vi "OEE_SCREEN_1_recolor_init.vi"(7 "SCREEN_1_recolor_references":T1, 8 "error_in":errorcluster) -> (0 "error_out":errorcluster)   [LabVIEW 2019]
uses:
  typedef/SCREEN_1_recolor_references.ctl
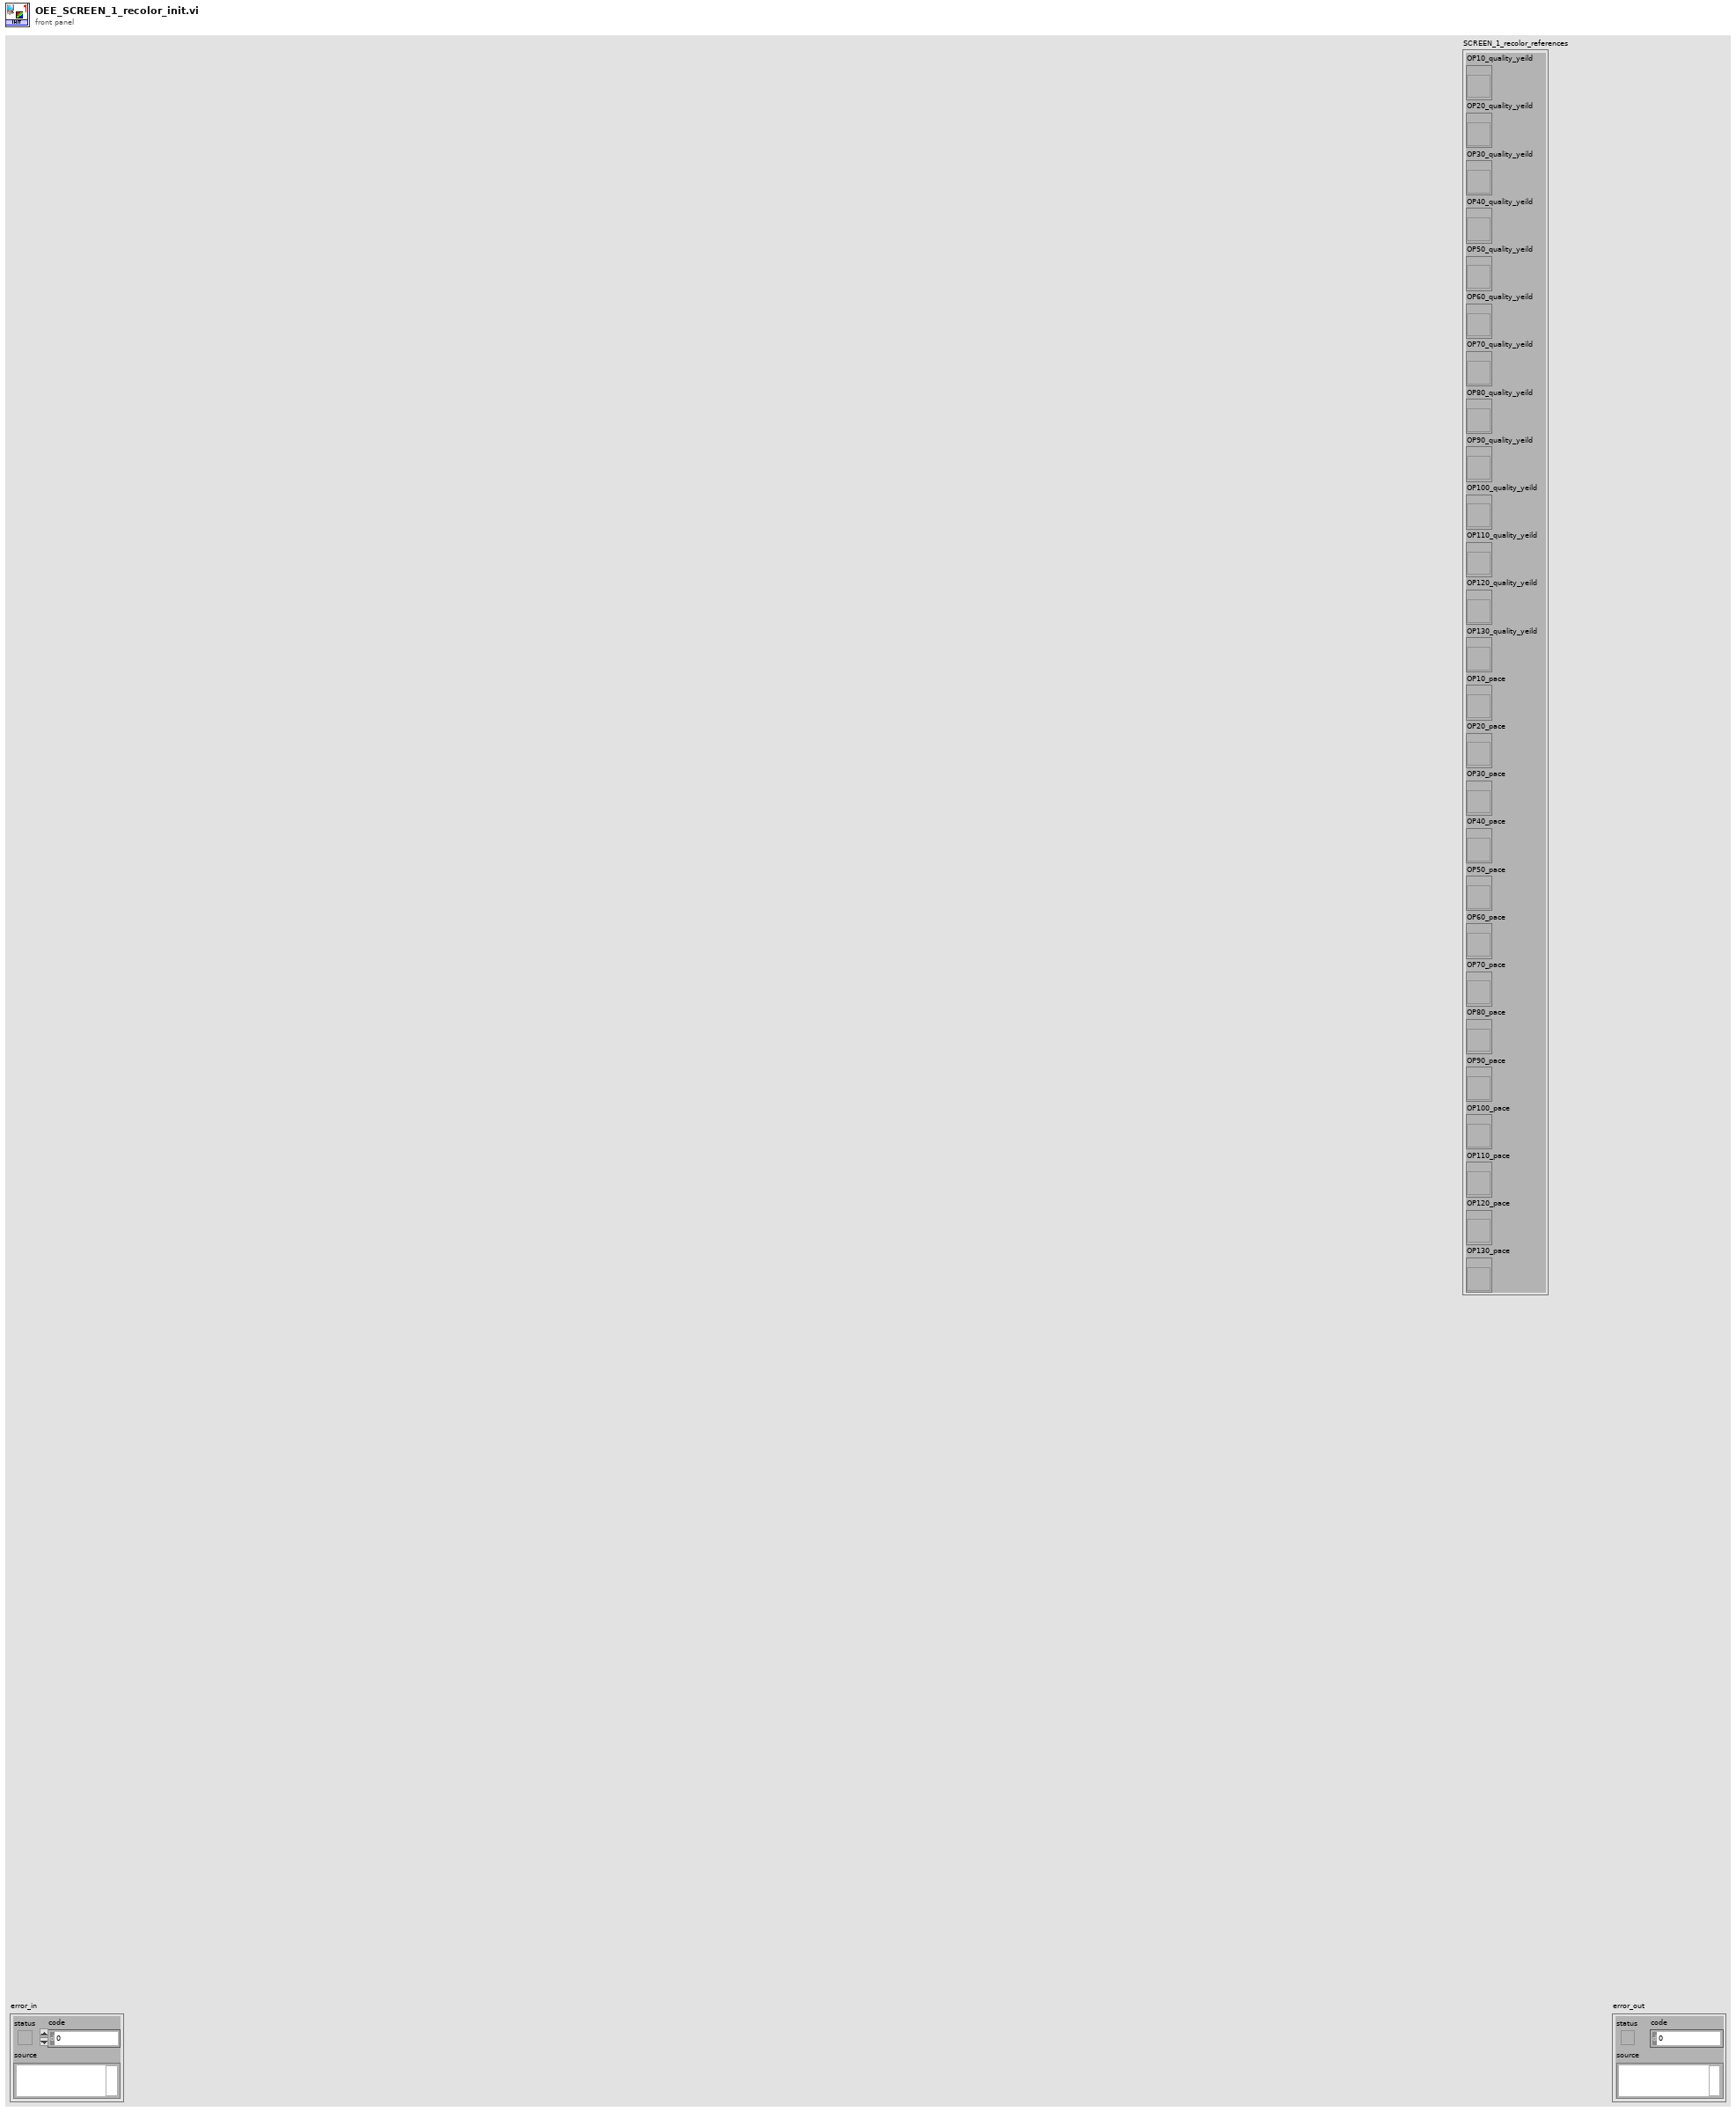
[diagram p1: front panel]
types:
  T1 = typedef "SCREEN_1_recolor_references.ctl" = cluster{"OP10_quality_yeild":refnum<vi>, "OP20_quality_yeild":refnum<vi>, "OP30_quality_yeild":refnum<vi>, "OP40_quality_yeild":refnum<vi>, "OP50_quality_yeild":refnum<vi>, "OP60_quality_yeild":refnum<vi>, "OP70_quality_yeild":refnum<vi>, "OP80_quality_yeild":refnum<vi>, "OP90_quality_yeild":refnum<vi>, "OP100_quality_yeild":refnum<vi>, "OP110_quality_yeild":refnum<vi>, "OP120_quality_yeild":refnum<vi>, "OP130_quality_yeild":refnum<vi>, "OP10_pace":refnum<vi>, "OP20_pace":refnum<vi>, "OP30_pace":refnum<vi>, "OP40_pace":refnum<vi>, "OP50_pace":refnum<vi>, "OP60_pace":refnum<vi>, "OP70_pace":refnum<vi>, "OP80_pace":refnum<vi>, "OP90_pace":refnum<vi>, "OP100_pace":refnum<vi>, "OP110_pace":refnum<vi>, "OP120_pace":refnum<vi>, "OP130_pace":refnum<vi>}
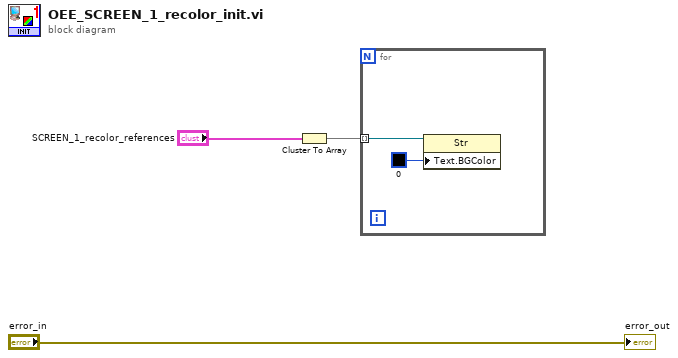
[diagram p0: block diagram]
diagram:
  n1 = Cluster To Array(cluster="SCREEN_1_recolor_references") -> (array=w1:refnum<vi>[])
  n2 = for {
    tunnel: w1 -> [w4] mode=indexing
    n3 = property class="Str"(reference=w4, "Text.BGColor"=u32 0) -> ()  [unwired: 1 in, 2 out]
  }
  "error_out" <- "error_in"
